vi "XBEE Rx Serial Frame Processor.vi"(6 "stop":bool, 9 "RX Frame Queue":refnum<queue>, 11 "VISA Serial Port":refnum<visa-resource-name>) -> (0 "Consumer error out":errorcluster, 1 "Producer error out":errorcluster)   [LabVIEW 2014]
uses:
  WiFi API Frame Type.ctl
  WiFi API Frame.ctl
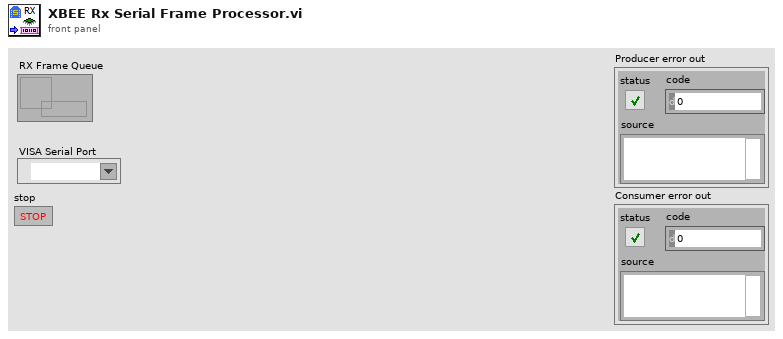
[diagram p1: front panel]
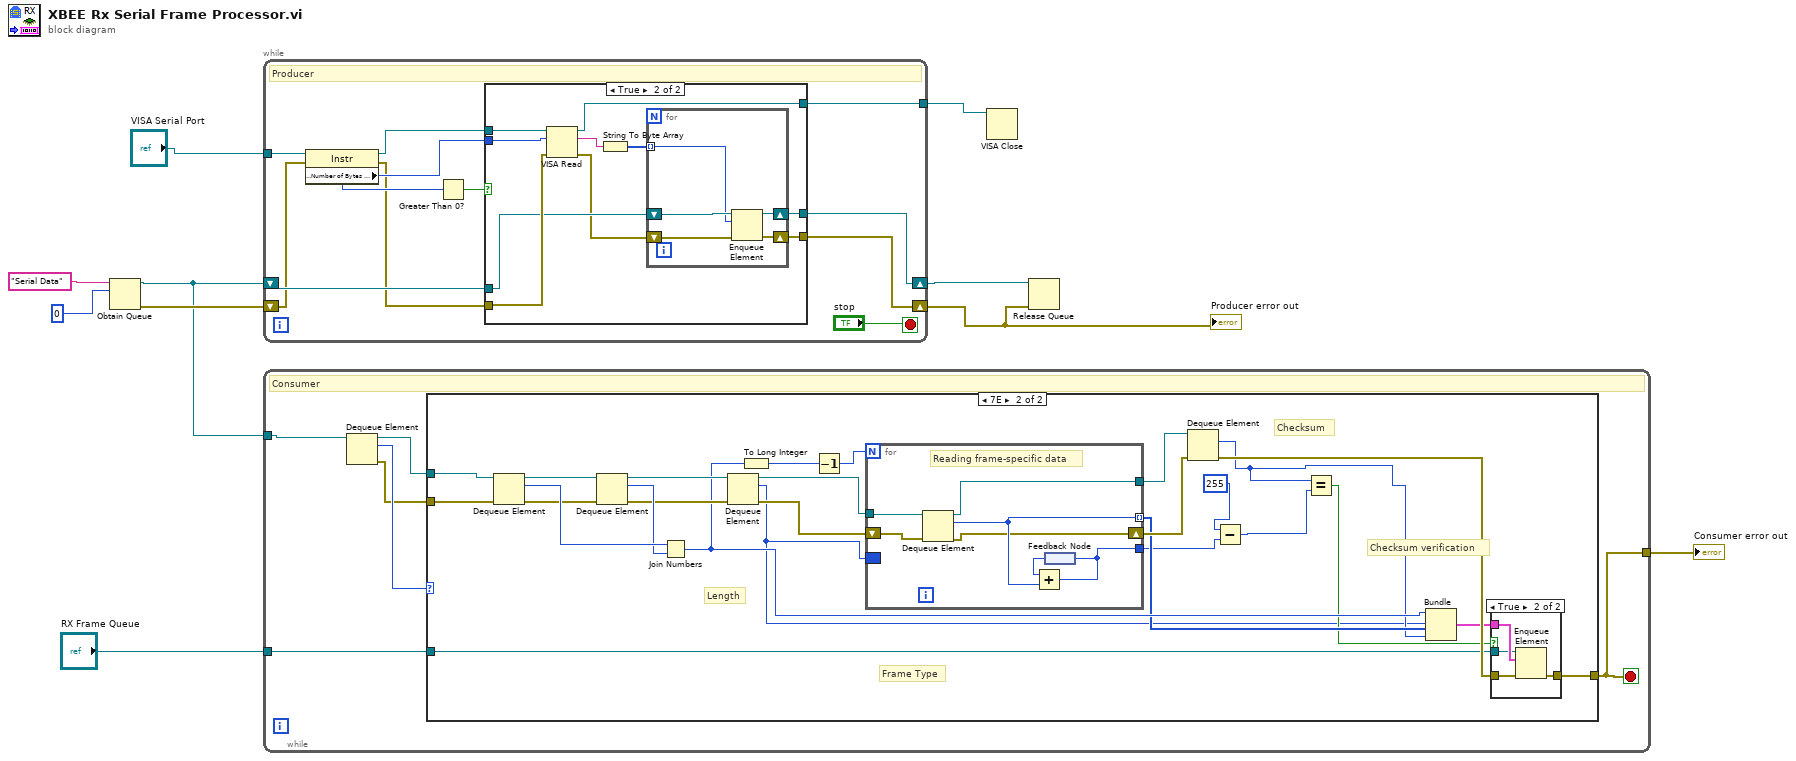
[diagram p0: block diagram]
diagram:
  n1 = Obtain Queue(name (unnamed)="Serial Data", element data type=u8 0) -> (queue out=w6:refnum<queue>, error out=w7:errorcluster)  [unwired: 3 in, 1 out]
  n2 = while {
    tunnel: "VISA Serial Port" -> [w21]
    shift-right: [w15] -> w5
    shift-left: w6 -> [w19]
    shift-right: [w14] -> w4
    shift-left: w7 -> [w12]
    tunnel: [w13] -> w2
    stop <- "stop" stop-if-true
    # "Producer"
    n3 = property class="Instr"(reference=w21, error in=w12) -> (reference out=w18:refnum<visa-resource-name>, error out=w11:errorcluster, "Serial Settings:Number of Bytes at Serial Port"=w17:u32)
    n4 = Greater Than 0?(x=w17) -> (x > 0?=w20:bool)
    n5 = case shown="True" w20 {
      tunnel: w19 -> [w24 w29]
      tunnel: w18 -> [w22 w34]
      tunnel: w17 -> [_ w33]
      tunnel: w11 -> [w23 w31]
      tunnel: [w24 w28] -> w15
      tunnel: [w23 w27] -> w14
      tunnel: [w22 w25] -> w13
      frame False {
      }
      frame True {
        n6 = VISA Read(VISA resource name=w34, byte count=w33, error in (no error)=w31) -> (VISA resource name out=w25:refnum<visa-resource-name>, read buffer=w32:string, error out=w26:errorcluster)  [unwired: 1 out]
        n7 = String To Byte Array(string=w32) -> (unsigned byte array=w30:u8[])
        n8 = for {
          tunnel: w30 -> [w38] mode=indexing
          shift-right: [w37] -> w28
          shift-left: w29 -> [w39]
          shift-right: [w36] -> w27
          shift-left: w26 -> [w35]
          n9 = Enqueue Element(queue=w39, element=w38, error in (no error)=w35) -> (queue out=w37:refnum<queue>, error out=w36:errorcluster)  [unwired: 1 in, 1 out]
        }
      }
    }
  }
  "Producer error out" <- w4
  n10 = while {
    tunnel: w6 -> [w45]
    tunnel: [w41] -> w3
    tunnel: "RX Frame Queue" -> [w40]
    stop <- w41 stop-if-true
    # "Consumer"
    n11 = Dequeue Element(queue=w45) -> (queue out=w44:refnum<queue>, element=w43:u8, error out=w42:errorcluster)  [unwired: 2 in, 1 out]
    n12 = case shown="7E" w43 {
      tunnel: w44 -> [_ w72]
      tunnel: w42 -> [w46 w61]
      tunnel: w40 -> [_ w53]
      tunnel: [w46 w55] -> w41
      frame 0, Default {
      }
      frame 126 {
        # "Checksum"
        # "Length"
        # "Checksum verification"
        # "Frame Type"
        n13 = Dequeue Element(queue=w72, error in (no error)=w61) -> (queue out=w71:refnum<queue>, element=w70:u8, error out=w62:errorcluster)  [unwired: 1 in, 1 out]
        n14 = Dequeue Element(queue=w71, error in (no error)=w62) -> (queue out=w68:refnum<queue>, element=w69:u8, error out=w63:errorcluster)  [unwired: 1 in, 1 out]
        n15 = Join Numbers(hi=w70, lo=w69) -> ((hi.lo)=w58:u16)
        n16 = Dequeue Element(queue=w68, error in (no error)=w63) -> (queue out=w67:refnum<queue>, element=w47:u8, error out=w64:errorcluster)  [unwired: 1 in, 1 out]
        n17 = To Long Integer(number=w58) -> (32bit integer=w65:i32)
        n18 = Decrement(x=w65) -> (x-1=w66:i32)
        n19 = for {
          N: w66 -> [_]
          tunnel: w67 -> [w84]
          tunnel: [w80] -> w57 mode=indexing
          tunnel: [w82] -> w60
          tunnel: [w81] -> w50
          shift-right: [w78] -> w59
          shift-left: w64 -> [w83]
          border: w47 -> [_]
          # "Reading frame-specific data"
          n20 = Dequeue Element(queue=w84, error in (no error)=w83) -> (queue out=w82:refnum<queue>, element=w80:u8, error out=w78:errorcluster)  [unwired: 1 in, 1 out]
          n21 = feedback #1() -> (w79:u8)
          n22 = Add(x=w79, y=w80) -> (x+y=w81:u8)
          n23 = feedback-in #1(w81) -> ()
        }
        n24 = Dequeue Element(queue=w60, error in (no error)=w59) -> (element=w49:u8, error out=w56:errorcluster)  [unwired: 1 in, 2 out]
        n25 = Subtract(x=u8 255, y=w50) -> (x-y=w48:u8)
        n26 = Equal?(x=w49, y=w48) -> (x = y?=w52:bool)
        n27 = Bundle(w58, w47, w57, w49) -> (w54:cluster{u16, u8, u8[], u8})  [unwired: 1 in]
        n28 = case shown="True" w52 {
          tunnel: w56 -> [w73 w77]
          tunnel: [w73 w76] -> w55
          tunnel: w54 -> [_ w75]
          tunnel: w53 -> [_ w74]
          frame False {
          }
          frame True {
            n29 = Enqueue Element(queue=w74, element=w75, error in (no error)=w77) -> (error out=w76:errorcluster)  [unwired: 1 in, 2 out]
          }
        }
      }
    }
  }
  "Consumer error out" <- w3
  n30 = VISA Close(VISA resource name=w2) -> ()  [unwired: 1 in, 1 out]
  n31 = Release Queue(queue=w5, error in (no error)=w4) -> ()  [unwired: 1 in, 3 out]
